vi "write flicker file.vi"(6 "Notes in":string, 7 "date/time string":timestamp, 8 "error in (no error)":errorcluster, 9 "Flicker Light Measurement":waveform(dbl), 10 "Flicker Dark Measurement":waveform(dbl), 11 "Metadata In":string[][](array[string])) -> (0 "error out":errorcluster)   [LabVIEW 2013]
uses:
  <vilib>/Waveform/WDTOps.llb/WDT Waveform Duration DBL.vi
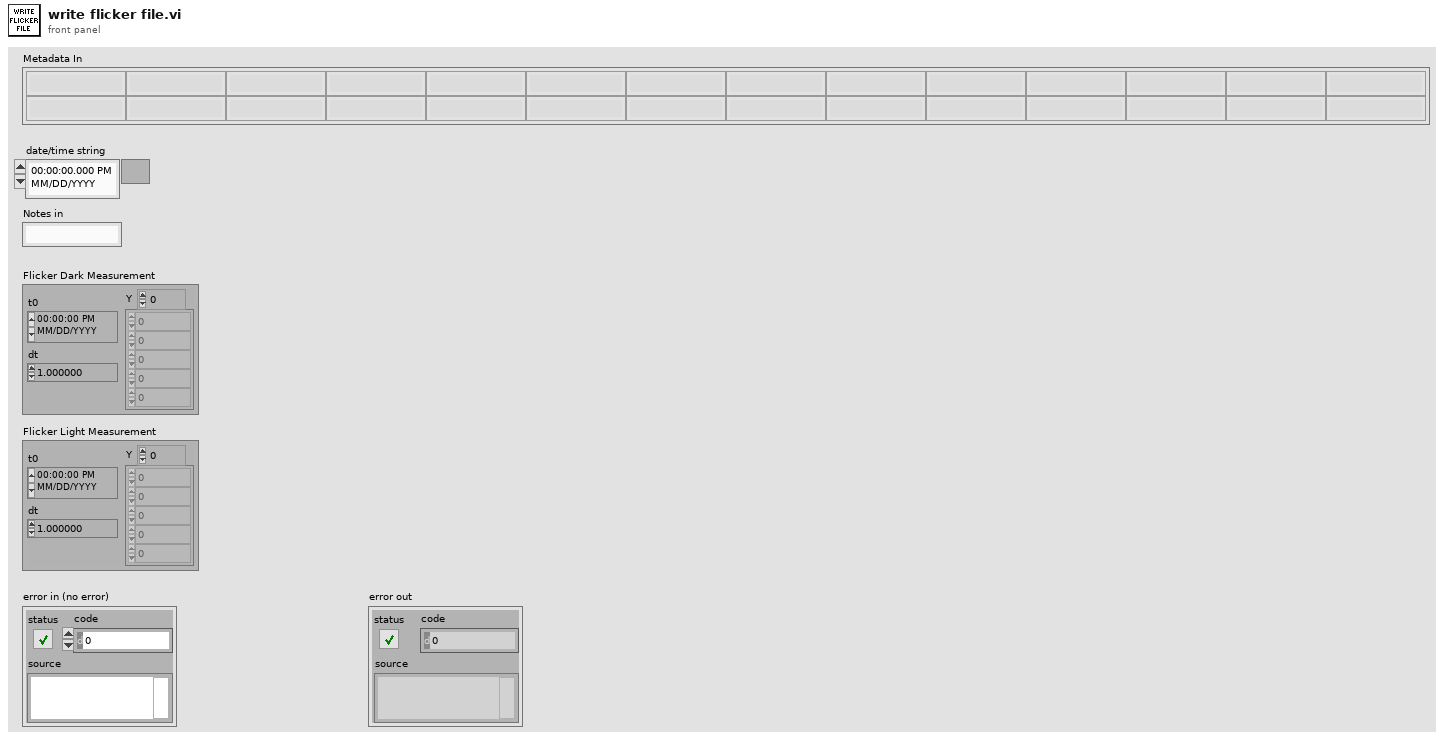
[diagram p1: front panel]
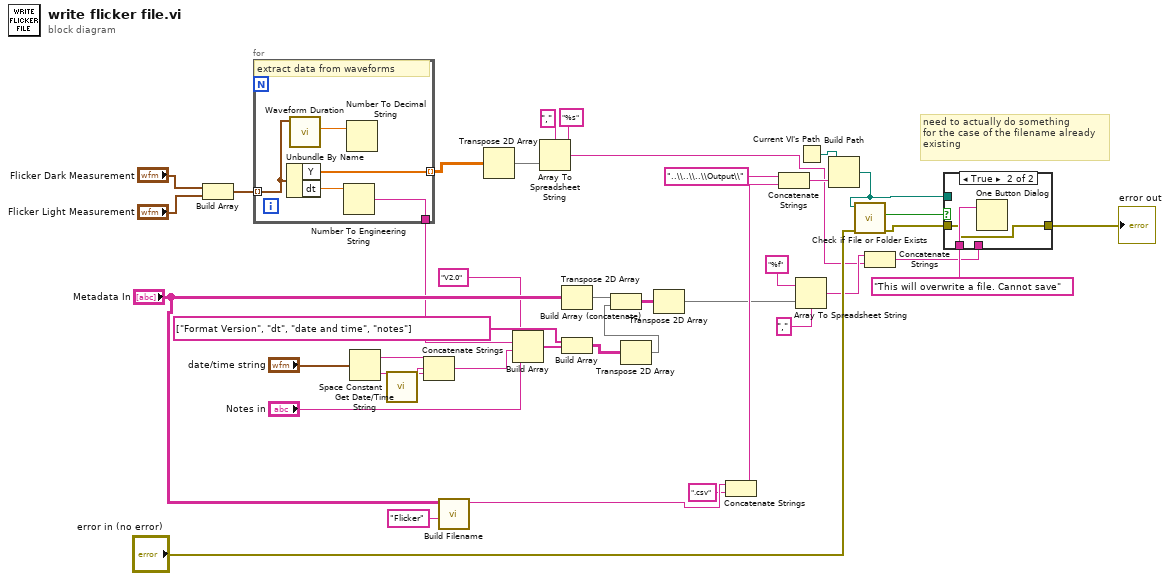
[diagram p0: block diagram]
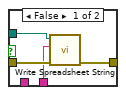
[diagram p2: hidden frame]
diagram:
  # "need to actually do something \nfor the case of the filename already\nexisting"
  n1 = Build Array("Flicker Dark Measurement", "Flicker Light Measurement") -> (w35:waveform(dbl)[])
  n2 = for {
    tunnel: w35 -> [w46] mode=indexing
    tunnel: [w45] -> w23
    tunnel: [w42] -> w8 mode=indexing
    # "extract data from waveforms"
    n3 = Unbundle By Name(w46) -> ("Y"=w42:dbl[], "dt"=w44:dbl)
    n4 = call-poly <vilib>:"Waveform Duration.vi"("waveform in"=w46) -> ("duration"=w43:dbl)  [unwired: 8 in, 2 out]
    n5 = Number To Engineering String(4:w44) -> (0:w45:string)  [unwired: 3 in]
    n6 = Number To Decimal String(number=w43) -> ()  [unwired: 1 in, 1 out]
  }
  n7 = Get Date/Time String(seconds (now)="date/time string") -> (date string=w3:string, time string=w2:string)  [unwired: 2 in]
  n8 = call <vilib>:"Space Constant.vi"() -> ("String"=w4:string)
  n9 = Concatenate Strings(w3, w4, w2) -> (w1:string)
  n10 = call "Build Filename.vi"("Measurment Type"="Flicker", "Metadata In"="Metadata In") -> ("String"=w39:string)  [unwired: 9 in]
  n11 = Transpose 2D Array(2D array=w8) -> (transposed array=w10:dbl[][])
  n12 = Build Array("V2.0" ("element"), w23, w1, "Notes in") -> (w20:string[])
  n13 = Array To Spreadsheet String(delimiter (Tab)=",", array=w10, 3:"%s" ("format string")) -> (spreadsheet string=w7:string)
  n14 = Transpose 2D Array(2D array="Metadata In") -> (transposed array=w28:string[][])
  n15 = Build Array(string[] ["Format Version", "dt", "date and time", "notes"], w20) -> (w13:string[][])
  n16 = Transpose 2D Array(2D array=w13) -> (transposed array=w12:string[][])
  n17 = Build Array (concatenate)(w28, w12) -> (w27:string[][])
  n18 = Transpose 2D Array(2D array=w27) -> (transposed array=w15:string[][])
  n19 = Concatenate Strings(w39, ".csv" ("string")) -> (w25:string)
  n20 = Concatenate Strings("..\\..\\..\\Output\\" ("name or relative path"), w25) -> (w24:string)
  n21 = Array To Spreadsheet String(delimiter (Tab)=",", array=w15, 3:"%f" ("format string")) -> (spreadsheet string=w17:string)
  n22 = Current VI's Path() -> (path=w31:path)
  n23 = Build Path(base path=w31, name or relative path=w24) -> (appended path=w30:path)
  n24 = call <vilib>:"Check if File or Folder Exists.vi"("error in (no error)"="error in (no error)", "path"=w30) -> ("error out"=w33:errorcluster, "file or folder exists?"=w41:bool)  [unwired: 7 in, 1 out]
  n25 = Concatenate Strings(w17, w7) -> (w16:string)
  n26 = case shown="True" w41 {
    tunnel: w30 -> [w50 _]
    tunnel: "This will overwrite a file. Cannot save" ("message") -> [_ w52]
    tunnel: w33 -> [w49 w51]
    tunnel: [w48 w51] -> w32
    tunnel: w16 -> [w47 _]
    frame False {
      n27 = call <vilib>:"Write Spreadsheet String.vi"("error in"=w49, "spreadsheet string"=w47, "file path (dialog if empty)"=w50) -> ("error out"=w48:errorcluster)  [unwired: 7 in, 1 out]
    }
    frame True {
      n28 = One Button Dialog(message=w52) -> ()  [unwired: 1 in, 1 out]
    }
  }
  "error out" <- w32
